vi "Check if configuration files exist.vi"(8 "error in (no error)":errorcluster, 11 "DAQOrcaFlashBase in":refnum<class "DAQOrcaFlash.lvclass">) -> (0 "error out":errorcluster, 2 "configuration file exists?":bool, 3 "DAQOrcaFlashBase out":refnum<class "DAQOrcaFlash.lvclass">)   [LabVIEW 2012, in "DAQOrcaFlash.lvclass"]
doc: "Checks whether all required configuration files for the component exist."
uses:
  DAQOrcaFlash.lvclass
  <vilib>/Distrio/Murmex/Murmex/Murmex.lvclass
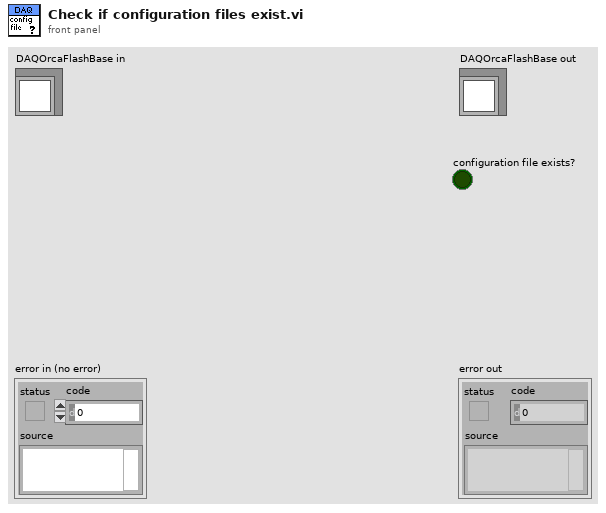
[diagram p1: front panel]
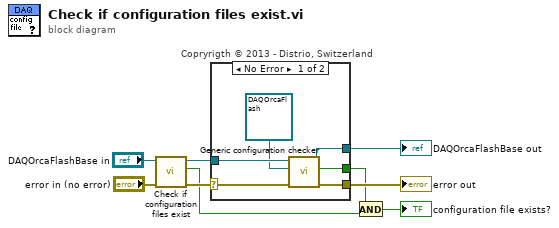
[diagram p0: block diagram]
diagram:
  n1 = call-parent "Check if configuration files exist.vi"("error in (no error)"="error in (no error)", "MurmexBase in"="DAQOrcaFlashBase in") -> ("error out"=w6:errorcluster, "configuration file exists?"=w2:bool, "MurmexBase out"=w7:refnum<class "DAQOrcaFlash.lvclass">)  [unwired: 7 in]
  n2 = case "Copryrigth © 2013 - Distrio, Switzerland" shown="No Error" w6 {
    selector: w6 -> [w15 w17]
    tunnel: [w13 w17] -> w5
    tunnel: [w11 w16] -> w4
    tunnel: w7 -> [w14 w16]
    tunnel: [w12 _] -> w3
    frame No Error {
      n3 = call <vilib>:"Generic configuration checker.vi"("error in (no error)"=w15, "inheritance level"=refnum<class "DAQOrcaFlash.lvclass"> refnum ("DAQOrcaFlash.lvclass"), "Murmex in"=w14) -> ("error out"=w13:errorcluster, "configuration file exists?"=w12:bool, "Murmex out"=w11:refnum<class "DAQOrcaFlash.lvclass">)  [unwired: 6 in]
    }
    frame Error {
    }
  }
  "error out" <- w5
  "DAQOrcaFlashBase out" <- w4
  n4 = And(x=w3, y=w2) -> (x .and. y?=→"configuration file exists?":bool)
